vi "Basic.vi"() -> ()   [LabVIEW 2018]
uses:
  <vilib>/userdefined/Silver/nirio_resource_slv.ctl
  Digitizer Control Class/Public/Acq Start Trigger Type.ctl
  <instrlib>/FlexRIO/API/Host/v1/NI FlexRIO/API/Reference Clock Source.ctl
  <instrlib>/FlexRIO/API/Host/v1/NI FlexRIO/API/Configure Reference Clock.vi
  <instrlib>/FlexRIO/API/Host/v1/NI FlexRIO API v1.lvlib
  Digitizer Control Class/Digitizer Control.lvclass
panel:
  out "Actual AI Offset (V)":dbl[](array[numeric]) format="%#_6p"
  in  "Desired AI Offset (V)":dbl[](array[numeric])=[0.0, 0.0] format="%#_6p"
  out "Actual AI Range (V)":dbl[](array[numeric]) format="%#_6p"
  in  "Desired AI Range (V)":dbl[](array[ring])=[1.0, 1.0] items=["200mV"=0.2, "1V"=1.0]
  out "Actual Digital Gain (dB)":dbl[](array[numeric]) format="%#_6p"
  out "Actual Digital Offset (V)":dbl[](array[numeric]) format="%#_6p"
  in  "Desired Digital Gain (dB)":dbl[](array[numeric])=[0.0, 0.0] format="%#_6p"
  in  "Desired Digital Offset (V)":dbl[](array[numeric])=[0.0, 0.0] format="%#_6p"
  in  "Enable Bit Packing":bool[](array[boolean])=[FALSE, FALSE]
  in  "digital high level?":bool=TRUE
  in  "trigger type":T1
  in  "analog trigger channel":string="AI0"
  in  "analog/digital rising edge?":bool=TRUE
  in  "analog level (V)":dbl format="%#_3p"
  in  "analog hysteresis (V)":dbl format="%#_3p"
  in  "digital trigger source":string(combo)="DIO"
  out "Acq Overflow":bool[](array[boolean])
  out "Error Out":errorcluster
  in  "Acq Update":bool
  in  "Desired Sampling Rate":dbl=800000000.0 format="%0.2p"
  in  "reference clock source":T2 items=["Default", "Onboard", "PXI_Clk10", "External", "None", "Baseboard Reference"]
  out "Actual Sampling Rate":dbl format="%#_6p"
  in  "Acq # of samples":i64[](array[numeric])=[100000, 100000]
  in  "AI channel":string="AI0,AI1"
  out "Device Power":dbl(slide) scale=-1.0..58.0 scale format="%#_3p"
  out "FPGA Temperature":dbl(slide) scale=0.0..100.0 scale format="%#_3p"
  in  "stop":bool
  in  "Waveform Tab Control":T3(tab)
  out "Waveform Graph":waveform(dbl)[](graph)
  out "Power Spectrum":cluster{"f0":dbl, "df":dbl, "magnitude":dbl[]}[](graph) caption="Waveform Graph"
  out "Limit (W)":dbl
  out "Power (W)":dbl
  out "Limit (C)":dbl
  out "Temp (C)":dbl format="%#_4p"
  in  "RIO Device":T4
  # "Overview: Acquisition with the transfer of the acquired waveform to the host.\nRequirements: PXIe-5774 (KU060)\nInstructions: \n 1. Select the RIO Device that corresponds to the FlexRIO target. \n 2. Optionally configure the clocking, trigger and acquisition configurations. \n 3. Run the VI"
  # "Acquisition Trigger"
  # "Clocking configuration"
  # "Acquisition Configuration"
  # "Digital Gain / Offset"
  # "Device Monitoring"
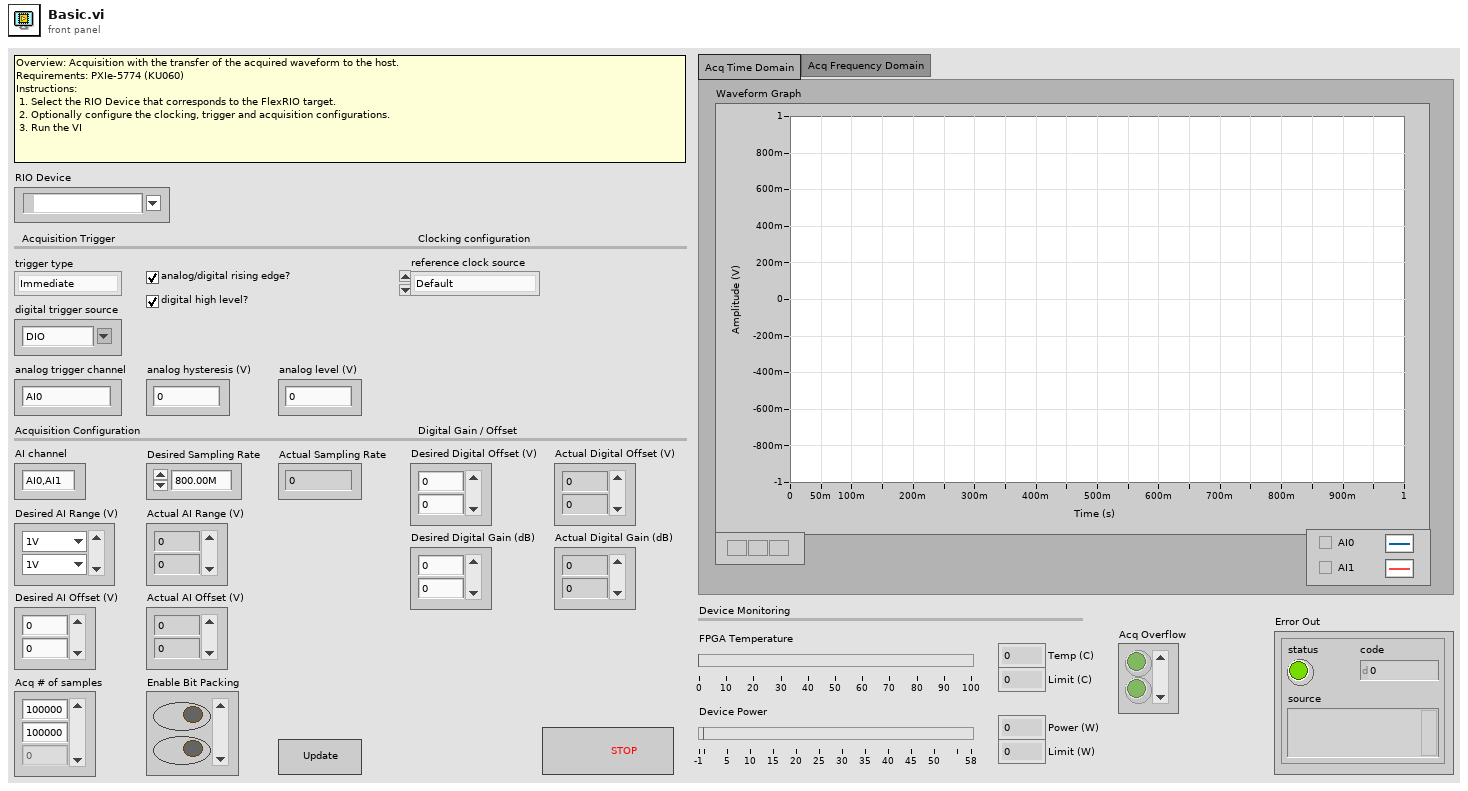
[diagram p1: front panel]
types:
  T1 = typedef "Digitizer Control.lvclass/Acq Start Trigger Type.ctl" = enum16{"Immediate", "Analog", "Digital Edge", "Digital Level"}
  T2 = typedef "NI FlexRIO API v1.lvlib/Reference Clock Source.ctl" = i32
  T3 = enum32{"Acq Time Domain", "Acq Frequency Domain"}
  T4 = typedef "nirio_resource_slv.ctl" = tag
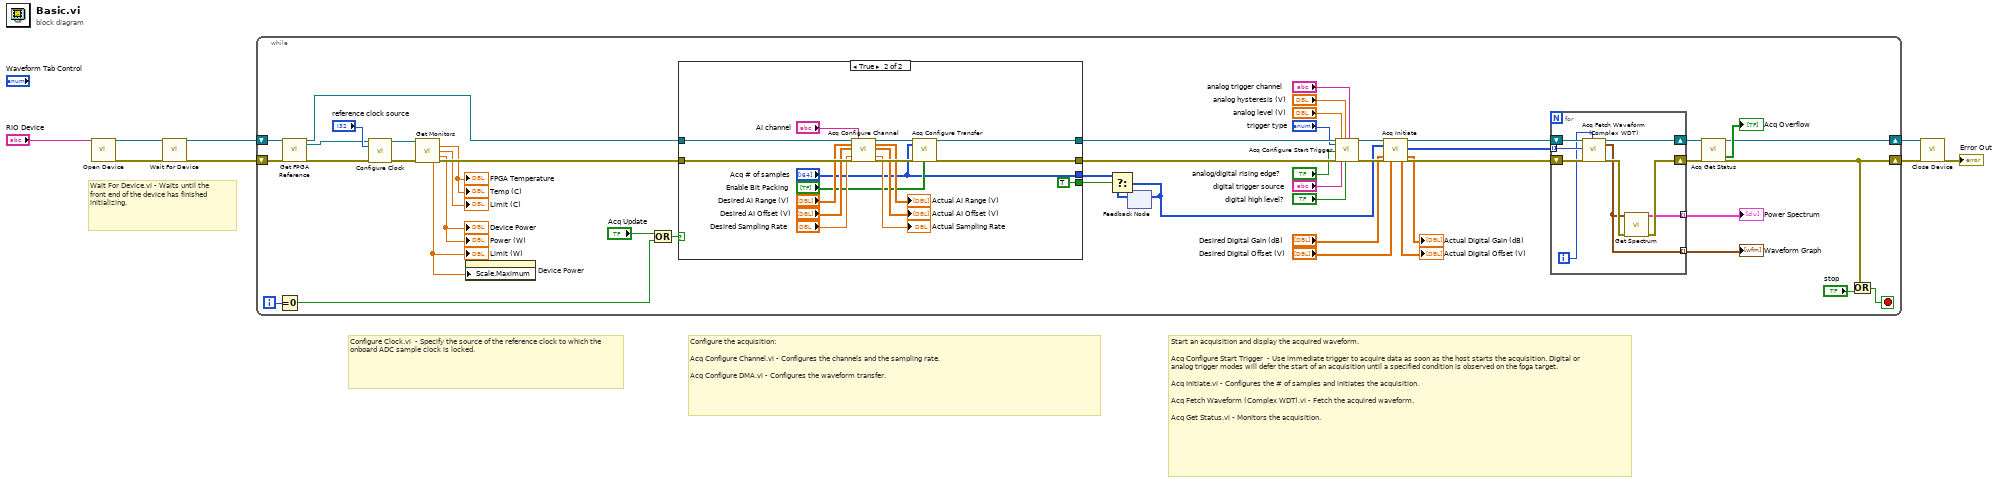
[diagram p0: block diagram]
diagram:
  # "Start an acquisition and display the acquired waveform.\n\nAcq Configure Start Trigger  - Use immediate trigger to acquire data as soon as the host starts the acquisition. Digital or analog trigger modes will defer the start of an acquisition until a specified condition is observed on the fpga target. \n\nAcq Initiate.vi - Configures the # of samples and initiates the acquisition.\n\nAcq Fetch Waveform (Complex WDT).vi - Fetch the acquired waveform.\n\nAcq Get Status.vi - Monitors the acquisition."
  # "Configure the acquisition:\n\nAcq Configure Channel.vi - Configures the channels and the sampling rate.\n\nAcq Configure DMA.vi - Configures the waveform transfer."
  # "Configure Clock.vi  - Specify the source of the reference clock to which the onboard ADC sample clock is locked."
  # "Wait For Device.vi - Waits until the front end of the device has finished initializing."
  n1 = call "Open Device.vi"("resource name"="RIO Device") -> ("session out"=w4:refnum<class "Digitizer Control.lvclass">, "error out"=w5:errorcluster)  [unwired: 17 in]
  n2 = call "Wait For Device.vi"("session in"=w4, "error in (no error)"=w5) -> ("session out"=w3:refnum<class "Digitizer Control.lvclass">, "error out"=w2:errorcluster)  [unwired: 15 in, 1 out]
  n3 = while {
    shift-right: [w10] -> w8
    shift-left: w2 -> [w29]
    shift-right: [w9] -> w6
    shift-left: w3 -> [w28]
    i -> [w39]
    stop <- w18 stop-if-true
    n4 = Equal To 0?(x=w39) -> (x = 0?=w41:bool)
    n5 = call "Get FPGA Reference.vi"("session in"=w28, "error in (no error)"=w29) -> ("session out"=w19:refnum<class "Digitizer Control.lvclass">, "fpga reference"=w27:refnum<k20>, "error out"=w50:errorcluster)  [unwired: 15 in]
    n6 = call-poly <instrlib>:"Configure Clock.vi"("fpga interface in"=w27, "reference clock source"="reference clock source", "error in"=w50) -> ("fpga interface out"=w43:refnum<k20>, "error out"=w51:errorcluster)  [unwired: 11 in]
    n7 = call "Get Monitors.vi"("fpga interface in"=w43, "error in (no error)"=w51) -> ("FPGA Temperature (C)"=→"Temp (C)" →"FPGA Temperature":dbl, "Temperature Limit (C)"=→"Limit (C)":dbl, "Total Power (W)"=→"Power (W)" →"Device Power":dbl, "Power Limit (W)"=w47:dbl, "error out"=w56:errorcluster)  [unwired: 8 in, 1 out]
    "Limit (W)" <- w47
    n8 = property on="Device Power" class="Slide (strict)"("Scale.Maximum"=w47) -> ()  [unwired: 2 in, 2 out]
    n9 = Or(x="Acq Update", y=w41) -> (x .or. y?=w40:bool)
    n10 = case shown="True" w40 {
      tunnel: w56 -> [w67 w82]
      tunnel: w19 -> [w66 w81]
      tunnel: [w67 w74] -> w53
      tunnel: [w66 w75] -> w55
      tunnel: [_ TRUE] -> w33
      tunnel: [_ "Acq # of samples"] -> w34
      frame False {
      }
      frame True {
        n11 = call "Acq Configure Channel.vi"("session in"=w81, "desired AI range (V)"="Desired AI Range (V)", "desired AI offset (V)"="Desired AI Offset (V)", "sampling rate (SPS)"="Desired Sampling Rate", "error in (no error)"=w82, "AI channel"="AI channel") -> ("session out"=w76:refnum<class "Digitizer Control.lvclass">, "actual AI range (V)"=→"Actual AI Range (V)":dbl[], "actual AI offset (V)"=→"Actual AI Offset (V)":dbl[], "actual sampling rate (SPS)"=→"Actual Sampling Rate":dbl, "error out"=w83:errorcluster)  [unwired: 7 in, 2 out]
        n12 = call "Acq Configure Transfer.vi"("session in"=w76, "host DMA buffer size (samples)"="Acq # of samples", "error in (no error)"=w83, "enable bit packing (F)"="Enable Bit Packing") -> ("session out"=w75:refnum<class "Digitizer Control.lvclass">, "error out"=w74:errorcluster)  [unwired: 9 in, 5 out]
      }
    }
    n13 = feedback #1() -> (w31:i64[])  [unwired: 1 in]
    n14 = Select(t=w34, s=w33, f=w31) -> (s? t:f=w32:i64[])
    n15 = feedback-in #1(w32) -> ()
    n16 = call "Acq Configure Start Trigger.vi"("session in"=w55, "trigger type (Immediate)"="trigger type", "rising edge? (T)"="analog/digital rising edge?", "error in (no error)"=w53, "analog level (0)"="analog level (V)", "digital trigger source (PXI_Trig0)"="digital trigger source", "analog hysteresis (0)"="analog hysteresis (V)", "digital high level? (T)"="digital high level?", "analog trigger channel (AI0)"="analog trigger channel") -> ("session out"=w54:refnum<class "Digitizer Control.lvclass">, "error out"=w52:errorcluster)  [unwired: 9 in]
    n17 = call "Acq Initiate.vi"("session in"=w54, "sample count (-1)"=w32, "desired digital gain (dB)"="Desired Digital Gain (dB)", "error in (no error)"=w52, "desired digital offset (V)"="Desired Digital Offset (V)") -> ("actual digital offset (V)"=→"Actual Digital Offset (V)":dbl[], "session out"=w30:refnum<class "Digitizer Control.lvclass">, "elements to read"=w11:i64[], "actual digital gain (dB)"=→"Actual Digital Gain (dB)":dbl[], "error out"=w38:errorcluster)  [unwired: 8 in, 2 out]
    n18 = for {
      tunnel: [w58] -> w37 mode=indexing
      tunnel: [w62] -> w36 mode=indexing
      shift-right: [w64] -> w13
      shift-left: w38 -> [w63]
      shift-right: [w60] -> w12
      shift-left: w30 -> [w61]
      tunnel: w11 -> [w59] mode=indexing
      i -> [w57]
      n19 = call "Acq Fetch Waveform (Complex WDT).vi"("session in"=w61, "elements to read"=w59, "error in (no error)"=w63, "channel index"=w57) -> ("session out"=w60:refnum<class "Digitizer Control.lvclass">, "waveform (V)"=w58:waveform(dbl), "error out"=w65:errorcluster)  [unwired: 11 in, 2 out]
      n20 = call "Get Spectrum.vi"("waveform (V)"=w58, "error in (no error)"=w65) -> ("power spectrum (dBm)"=w62:cluster{"f0":dbl, "df":dbl, "magnitude":dbl[]}, "error out"=w64:errorcluster)  [unwired: 12 in]
    }
    "Waveform Graph" <- w37
    "Power Spectrum" <- w36
    n21 = call "Acq Get Status.vi"("session in"=w12, "error in (no error)"=w13) -> ("session out"=w9:refnum<class "Digitizer Control.lvclass">, "overflow"=→"Acq Overflow":bool[], "error out"=w10:errorcluster)  [unwired: 8 in, 7 out]
    n22 = Or(x=w10, y="stop") -> (x .or. y?=w18:bool)
  }
  n23 = call "Close Device.vi"("session in"=w6, "error in (no error)"=w8) -> ("error out"=→"Error Out":errorcluster)  [unwired: 17 in]
